vi "Constructor.vi"(8 "error in (no error)":errorcluster, 11 "RunningAverageCalculation in":refnum<class "RunningAverageCalculation.lvclass">) -> (0 "error out":errorcluster, 3 "RunningAverageCalculation out":refnum<class "RunningAverageCalculation.lvclass">)   [LabVIEW 2015, in "RunningAverageCalculation.lvclass"]
uses:
  Waveform-Processing-Custom-Device Configuration.llb/RunningAverageCalculation.lvclass
  Waveform-Processing-Custom-Device Configuration.llb/WaveformCalculation.lvclass/WaveformCalculation.ctl
  Waveform-Processing-Custom-Device Configuration.llb/WaveformCalculation.lvclass
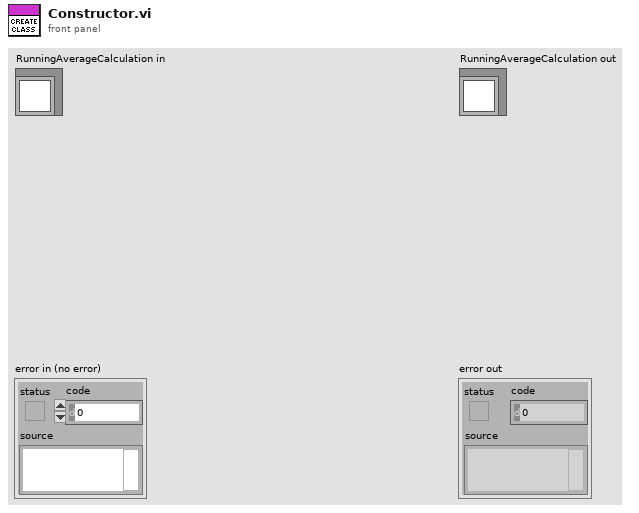
[diagram p1: front panel]
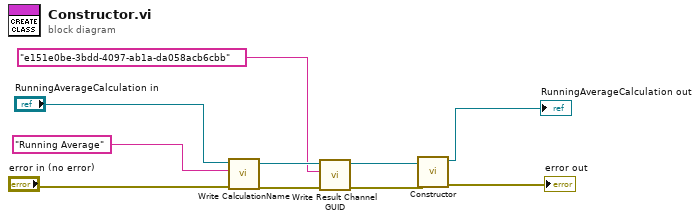
[diagram p0: block diagram]
diagram:
  n1 = call "Write CalculationName.vi"("error in (no error)"="error in (no error)", "CalculationName"="Running Average", "WaveformCalculation in"="RunningAverageCalculation in") -> ("error out"=w5:errorcluster, "WaveformCalculation out"=w2:refnum<class "RunningAverageCalculation.lvclass">)  [unwired: 7 in]
  n2 = call "Write Result Channel GUID.vi"("error in (no error)"=w5, "Result Channel GUID"="e151e0be-3bdd-4097-ab1a-da058acb6cbb", "WaveformCalculation in"=w2) -> ("error out"=w4:errorcluster, "WaveformCalculation out"=w3:refnum<class "RunningAverageCalculation.lvclass">)  [unwired: 7 in]
  n3 = call-parent "Constructor.vi"("error in (no error)"=w4, "WaveformCalculation in"=w3) -> ("error out"=→"error out":errorcluster, "WaveformCalculation out"=→"RunningAverageCalculation out":refnum<class "RunningAverageCalculation.lvclass">)  [unwired: 8 in]
